vi "Initialize Waveform Page.vi"(8 "error in":errorcluster, 11 "Node Ptr":T1 format="%.0x") -> (0 "error out":errorcluster, 2 "Waveform Settings Table":string[][](array[string]), 3 "Node Ptr out":T1=18446744073709551615 format="%.0x")   [LabVIEW 2026]
uses:
  <vilib>/NI VeriStand/Custom Device API/Custom Device Item Ref.ctl
  <vilib>/NI VeriStand/Custom Device API/Custom Device API.lvlib
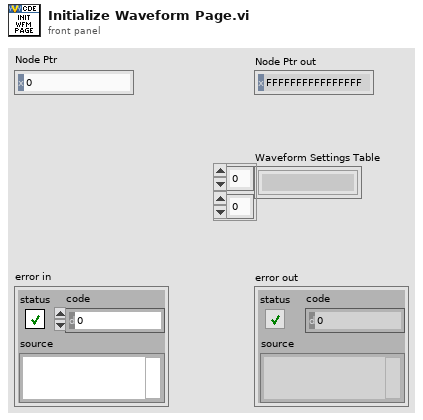
[diagram p1: front panel]
types:
  T1 = typedef "Custom Device API.lvlib/Custom Device Item Ref.ctl" = u64
  T2 = typedef "WaveformSettings.ctl" = cluster{"Units":string, "DataType":i32}
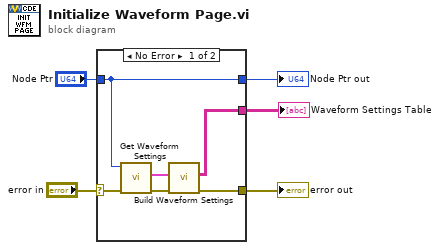
[diagram p0: block diagram]
diagram:
  n1 = case shown="No Error" "error in" {
    selector: "error in" -> [w10 w13]
    tunnel: "Node Ptr" -> [w8 w12]
    tunnel: [w9 w13] -> w3
    tunnel: [w7 _] -> w1
    tunnel: [w8 w12] -> w2
    frame No Error {
      n2 = call "Get Waveform Settings.vi"("error in"=w10, "Node Ptr"=w8) -> ("error out"=w11:errorcluster, "Waveform Settings"=w6:T2)  [unwired: 7 in, 1 out]
      n3 = call "Build Waveform Settings.vi"("error in"=w11, "Waveform Settings"=w6) -> ("error out"=w9:errorcluster, "Waveform Settings Table"=w7:string[][])  [unwired: 8 in]
    }
    frame Error {
    }
  }
  "error out" <- w3
  "Node Ptr out" <- w2
  "Waveform Settings Table" <- w1
